vi "Initialize.vi"(8 "error in (no error)":errorcluster, 11 "Object ref in":T1) -> (0 "error out":errorcluster, 3 "Object ref out":T1)   [LabVIEW 2013, in "SLMControl.lvlib" / "SC-Main.lvclass"]
uses:
  SC-Main.lvclass
  Object-reference.ctl
  Application-status.ctl
  UI/Control-names.ctl
  SC-Main.lvclass/SC-Main.ctl
  Read UI.vi
  UI/Set-control-boolean.vi
  UI/SC-UI.lvclass
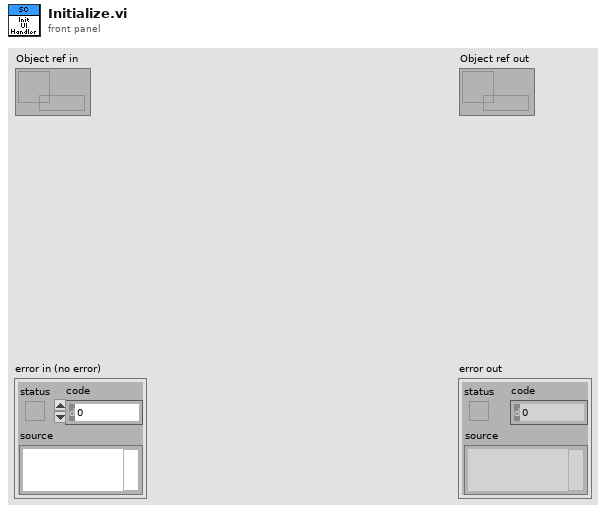
[diagram p1: front panel]
types:
  T1 = typedef "SLMControl.lvlib/SC-Main.lvclass/Object-reference.ctl" = refnum<data-value>
  T2 = typedef "SLMControl.lvlib/SC-UI.lvclass/Control-names.ctl" = enum16{"Com-in", "Com-out", "Help", "Status", "Load configuration", "Save configuration", "Load lasing files", "Load deposition files", "Clear", "Files", "Activate", "Execute", "Abort", "Options", "Current layer", "Current iteration", "Last elapsed time", "Deposition status", "Lasing job", "Status LEDs", "Exiting led", "Initialized led", "Files loaded led", "Activated led", "Executing led", "Deposition led", "Lasing job led", "Lasing led"}
  T3 = typedef "SLMControl.lvlib/SC-Main.lvclass/Application-status.ctl" = enum16{"Idle", "Initialized", "Configured", "Activated", "Started", "Paused", "Stopped", "Reset", "Error", "Exited"}
  T4 = typedef "SLMControl.lvlib/SC-UI.lvclass/Panes-reference.ctl" = refnum<data-value>
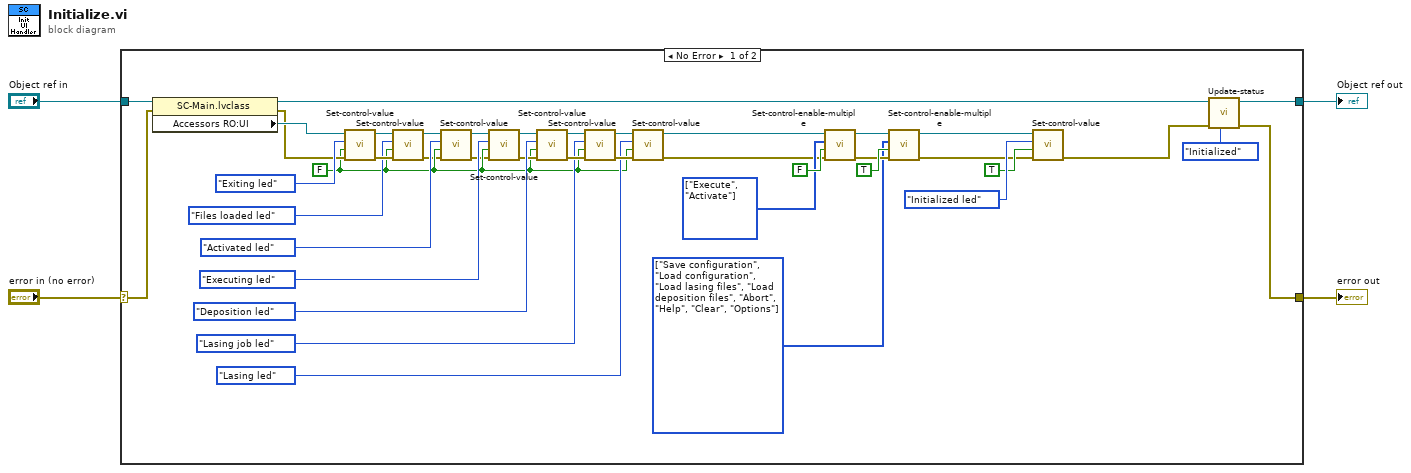
[diagram p0: block diagram]
diagram:
  n1 = case shown="No Error" "error in (no error)" {
    selector: "error in (no error)" -> [w29 w47]
    tunnel: [w44 w47] -> w3
    tunnel: [w43 w46] -> w1
    tunnel: "Object ref in" -> [w37 w46]
    frame No Error {
      w12 = T2[] [enum."Save configuration", enum."Load configuration", enum."Load lasing files", enum."Load deposition files", enum."Abort", enum."Help", enum."Clear", enum."Options"] items=["Com-in", "Com-out", "Help", "Status", "Load configuration", "Save configuration", "Load lasing files", "Load deposition files", "Clear", "Files", "Activate", "Execute", "Abort", "Options", "Current layer", "Current iteration", "Last elapsed time", "Deposition status", "Lasing job", "Status LEDs", "Exiting led", "Initialized led", "Files loaded led", "Activated led", "Executing led", "Deposition led", "Lasing job led", "Lasing led"] ("Control names")
      w13 = T2[] [enum."Execute", enum."Activate"] items=["Com-in", "Com-out", "Help", "Status", "Load configuration", "Save configuration", "Load lasing files", "Load deposition files", "Clear", "Files", "Activate", "Execute", "Abort", "Options", "Current layer", "Current iteration", "Last elapsed time", "Deposition status", "Lasing job", "Status LEDs", "Exiting led", "Initialized led", "Files loaded led", "Activated led", "Executing led", "Deposition led", "Lasing job led", "Lasing led"] ("Control names")
      w22 = FALSE
      n2 = property class="SC-Main.lvclass"(reference=w37, error in=w29) -> (reference out=w39:T1, error out=w30:errorcluster, "Accessors RO:UI"=w32:T4)
      n3 = call-poly "Set-control-value.vi"("error in (no error)"=w30, "Value"=w22, "Control name"=Control-names."Exiting led", "Panes in"=w32) -> ("error out"=w36:errorcluster, "Panes out"=w33:T4)  [unwired: 6 in]
      n4 = call-poly "Set-control-value.vi"("error in (no error)"=w36, "Value"=w22, "Control name"=Control-names."Files loaded led", "Panes in"=w33) -> ("error out"=w18:errorcluster, "Panes out"=w21:T4)  [unwired: 6 in]
      n5 = call-poly "Set-control-value.vi"("error in (no error)"=w18, "Value"=w22, "Control name"=Control-names."Activated led", "Panes in"=w21) -> ("error out"=w19:errorcluster, "Panes out"=w20:T4)  [unwired: 6 in]
      n6 = call-poly "Set-control-value.vi"("error in (no error)"=w19, "Value"=w22, "Control name"=Control-names."Executing led", "Panes in"=w20) -> ("error out"=w38:errorcluster, "Panes out"=w42:T4)  [unwired: 6 in]
      n7 = call-poly "Set-control-value.vi"("error in (no error)"=w38, "Value"=w22, "Control name"=Control-names."Deposition led", "Panes in"=w42) -> ("error out"=w27:errorcluster, "Panes out"=w28:T4)  [unwired: 6 in]
      n8 = call-poly "Set-control-value.vi"("error in (no error)"=w27, "Value"=w22, "Control name"=Control-names."Lasing job led", "Panes in"=w28) -> ("error out"=w25:errorcluster, "Panes out"=w24:T4)  [unwired: 6 in]
      n9 = call-poly "Set-control-value.vi"("error in (no error)"=w25, "Value"=w22, "Control name"=Control-names."Lasing led", "Panes in"=w24) -> ("error out"=w5:errorcluster, "Panes out"=w6:T4)  [unwired: 6 in]
      n10 = call "Set-control-enable-multiple.vi"("error in (no error)"=w5, "Enable?"=FALSE, "Control names"=w13, "Panes in"=w6) -> ("error out"=w14:errorcluster, "Panes out"=w17:T4)  [unwired: 6 in]
      n11 = call "Set-control-enable-multiple.vi"("error in (no error)"=w14, "Enable?"=TRUE, "Control names"=w12, "Panes in"=w17) -> ("error out"=w7:errorcluster, "Panes out"=w8:T4)  [unwired: 6 in]
      n12 = call-poly "Set-control-value.vi"("error in (no error)"=w7, "Value"=TRUE, "Control name"=Control-names."Initialized led", "Panes in"=w8) -> ("error out"=w9:errorcluster)  [unwired: 6 in, 1 out]
      n13 = call "Update-status.vi"("Status"=Application-status."Initialized", "error in (no error)"=w9, "Object ref in"=w39) -> ("error out"=w44:errorcluster, "Object ref out"=w43:T1)  [unwired: 7 in]
    }
    frame Error {
    }
  }
  "error out" <- w3
  "Object ref out" <- w1
